vi "Stop Acquisition.vi"(8 "error in (no error)":errorcluster, 11 "DAQ AI in":refnum<class "DAQ AI.lvclass">) -> (0 "error out":errorcluster, 3 "DAQ AI out":refnum<class "DAQ AI.lvclass">)   [LabVIEW 2020, in "DAQ AI.lvlib" / "DAQ AI.lvclass"]
uses:
  DAQ AI.lvclass
  <vilib>/ActorFramework/Time-Delayed Send Message/Time-Delay Override Options.ctl
  DAQ AI.lvclass/DAQ AI.ctl
  <vilib>/ActorFramework/Actor Framework.lvlib
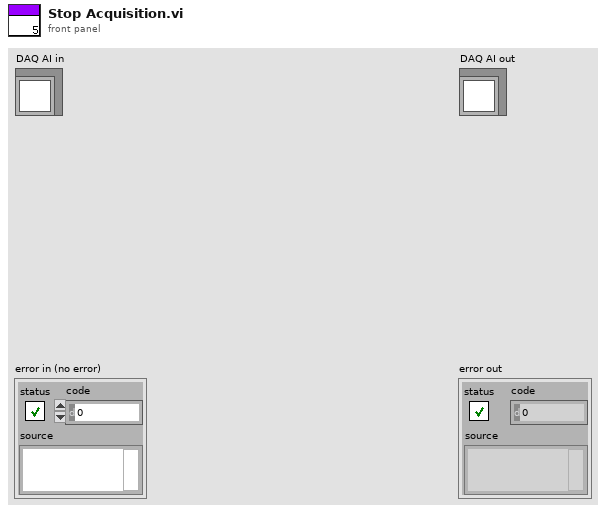
[diagram p1: front panel]
types:
  T1 = typedef "Actor Framework.lvlib/Time-Delay Override Options.ctl" = enum16{"Send next copy now", "Skip next scheduled copy", "Send next copy now and stop all further copies", "Stop all further copies"}
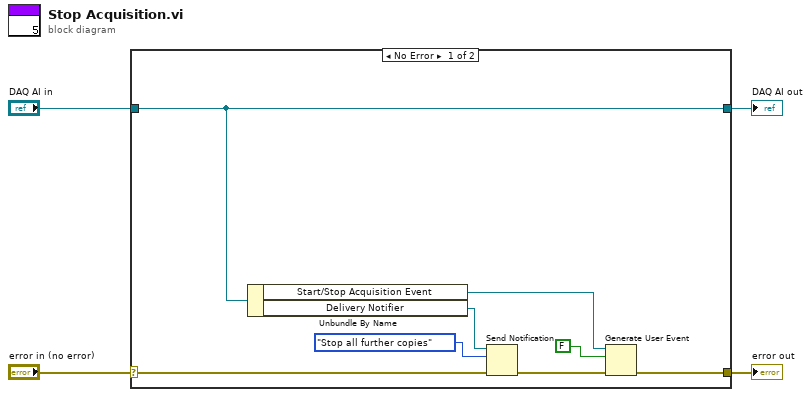
[diagram p0: block diagram]
diagram:
  n1 = case shown="No Error" "error in (no error)" {
    selector: "error in (no error)" -> [w6 w14]
    tunnel: [w9 w14] -> w3
    tunnel: [w10 w13] -> w1
    tunnel: "DAQ AI in" -> [w10 w13]
    frame No Error {
      n2 = Unbundle By Name(w10) -> ("Start/Stop Acquisition Event"=w12:refnum<user-event>, "Delivery Notifier"=w8:refnum<notifier>)
      n3 = Send Notification(notification=Time-Delay_Override_Options."Stop all further copies", notifier=w8, error in (no error)=w6) -> (error out=w5:errorcluster)  [unwired: 1 out]
      n4 = Generate User Event(user event=w12, event data cluster=FALSE ("event data"), error in=w5) -> (error out=w9:errorcluster)  [unwired: 1 in, 1 out]
    }
    frame Error {
    }
  }
  "error out" <- w3
  "DAQ AI out" <- w1
